vi "Mecanum Drive.vi"(0 "Division":dbl=1.0 format="%#_13g", 4 "Turning":dbl format="%#_13g", 5 "F/R":dbl, 6 "Strafing":dbl, 7 "State Control":enum16{"Open", "Run", "End"}(ring)) -> ()   [LabVIEW 2013]
doc: "Controls the Mecanum Drive. PWM ports are 1-4 counter-clockwise starting at the front-right motor.\n\nState Controls should be: \"Open\" in Begin.vi, \"Run\" in drive code, and \"End\" in Finish.vi. Motor Values are required for the \"Run\" state."
uses:
  <vilib>/Rock Robotics/SystemInterfaces/DIO/FPGA_DIOPWMChannel.ctl
  <vilib>/Rock Robotics/WPI/RobotDrive/WPI_RobotDriveOpen4MotorWithTalon.vi
  <vilib>/Rock Robotics/WPI/RobotDrive/WPI_RobotDriveMecanumDrive_Cartesian.vi
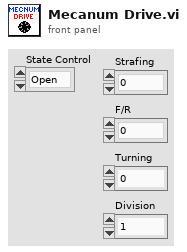
[diagram p1: front panel]
types:
  T1 = typedef "FPGA_DIOPWMChannel.ctl" = enum8{"PWM 1", "PWM 2", "PWM 3", "PWM 4", "PWM 5", "PWM 6", "PWM 7", "PWM 8", "PWM 9", "PWM 10", "Invalid"}
  T2 = typedef "WPI_RobotDriveDevRef.ctl" = cluster{"DevStatus":errorcluster, "Motors[]":T3[], "Square Inputs":bool, "Max Output":dbl, "Isochronous":bool}
  T3 = typedef "WPI_MotorControlDeviceRef.ctl" = cluster{"DeviceStatus":errorcluster, "Type":enum16{"PWM", "CAN"}, "PWM":cluster{"Digital Module":T4, "PWM Channel":T1, "DeadBand":T5}, "CAN":cluster{"Device Number":u8, "Control Mode":T6, "Semaphore":T7, "Max Vout":dbl}, "Invert":bool, "TransformRef":T8, "InvTransformRef":T8}
  T4 = typedef "FPGA_TypedefDigitalModule.ctl" = enum16{"Digital Module 1", "Digital Module 2"}
  T5 = typedef "WPI_PWMDeadband.ctl" = cluster{"Name":string, "maxPositivePwm":i32, "minPositivePwm":i32, "centerPwm":i32, "maxNegativePwm":i32, "minNegativePwm":i32, "angularRange":u16}
  T6 = typedef "WPI_CANJaguar_ControlMode.ctl" = enum8{"Percent VBus", "Current", "Speed", "Position", "Voltage"}
  T7 = typedef "Semaphore RefNum" = refnum<k1>
  T8 = typedef "WPI_PWMTransform_ConPane.ctl" = refnum<vi>
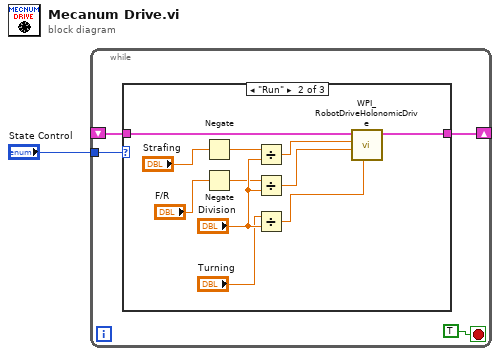
[diagram p0: block diagram]
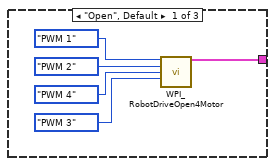
[diagram p2: hidden frame]
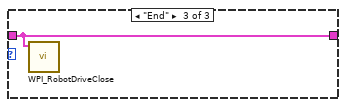
[diagram p3: hidden frame]
diagram:
  n1 = while {
    shift-right: [w5] -> _
    shift-left: _ -> [w4]
    tunnel: "State Control" -> [w3]
    stop <- TRUE stop-if-true
    n2 = case shown="\"Run\"" w3 {
      tunnel: [w10 w20 w22] -> w5
      tunnel: w4 -> [_ w21 w22]
      frame "Open", Default {
        n3 = call-poly <vilib>:"WPI_RobotDriveOpen4Motor.vi"("Rear Left Motor"=FPGA_DIOPWMChannel."PWM 1" ("PWMChannel"), "Rear Right Motor"=FPGA_DIOPWMChannel."PWM 2" ("PWMChannel"), "Front Left Motor"=FPGA_DIOPWMChannel."PWM 4" ("PWMChannel"), "Front Right Motor"=FPGA_DIOPWMChannel."PWM 3" ("PWMChannel")) -> ("RobotDriveDevRef"=w10:T2)  [unwired: 10 in, 1 out]
      }
      frame "Run" {
        n4 = Negate(x="Strafing") -> (-x=w12:dbl)
        n5 = Negate(x="F/R") -> (-x=w14:dbl)
        n6 = Divide(x=w12, y="Division") -> (x/y=w19:dbl)
        n7 = Divide(x=w14, y="Division") -> (x/y=w17:dbl)
        n8 = Divide(x="Turning", y="Division") -> (x/y=w16:dbl)
        n9 = call-poly <vilib>:"WPI_RobotDriveHolonomicDrive.vi"("Rotation"=w16, "Y"=w17, "X"=w19, "RobotDriveDevRef"=w21) -> ("RobotDriveDevRef"=w20:T2)  [unwired: 5 in, 2 out]
      }
      frame "End" {
        n10 = call <vilib>:"WPI_RobotDriveClose.vi"("RobotDriveDevRef"=w22) -> ()  [unwired: 10 in, 1 out]
      }
    }
  }
